vi "Initialize Hardware References.vi"(8 "error in (no error)":errorcluster, 9 "Relay Task Name":string, 10 "Vibration Task Name":string, 11 "Hardware Resources in":T1) -> (0 "error out":errorcluster, 3 "Hardware Resources out":T1)   [LabVIEW 2026, in "Acquisition.lvlib"]
doc: "Initialize the hardware references."
uses:
  Acquisition.lvlib
  Controls/Hardware Configuration.ctl
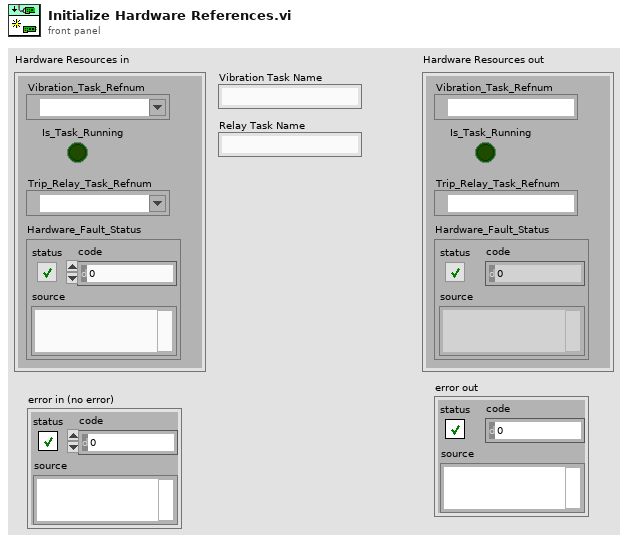
[diagram p1: front panel]
types:
  T1 = typedef "Acquisition.lvlib/Hardware Configuration.ctl" = cluster{"Vibration_Task_Refnum":refnum<k21>, "Is_Task_Running":bool, "Hardware_Fault_Status":errorcluster, "Trip_Relay_Task_Refnum":refnum<k21>}
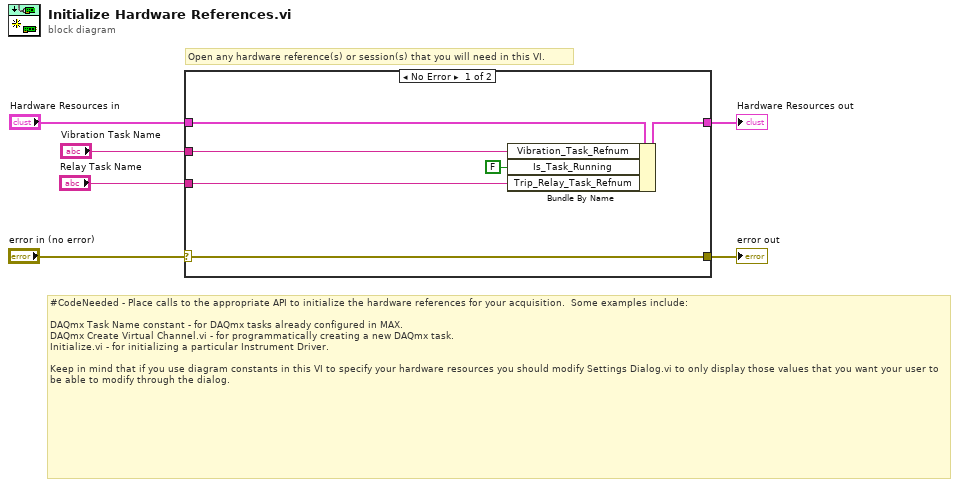
[diagram p0: block diagram]
diagram:
  # "Open any hardware reference(s) or session(s) that you will need in this VI."
  # "#CodeNeeded - Place calls to the appropriate API to initialize the hardware references for your acquisition.  Some examples include:\n\nDAQmx Task Name constant - for DAQmx tasks already configured in MAX.\nDAQmx Create Virtual Channel.vi - for programmatically creating a new DAQmx task.\nInitialize.vi - for initializing a particular Instrument Driver.\n\nKeep in mind that if you use diagram constants in this VI to specify your hardware resources you should modify Settings Dialog.vi to only display those values that you want your user to be able to modify through the dialog."
  n1 = case shown="No Error" "error in (no error)" {
    selector: "error in (no error)" -> [w11 w13]
    tunnel: [w11 w13] -> w5
    tunnel: "Hardware Resources in" -> [w10 w14]
    tunnel: [w12 w14] -> w3
    tunnel: "Vibration Task Name" -> [w9 _]
    tunnel: "Relay Task Name" -> [w7 _]
    frame No Error {
      n2 = Bundle By Name(cluster=w10, "Vibration_Task_Refnum"=w9, "Is_Task_Running"=FALSE, "Trip_Relay_Task_Refnum"=w7) -> (w12:T1)
    }
    frame Error {
    }
  }
  "Hardware Resources out" <- w3
  "error out" <- w5
